vi "__createNewRoom.vi"(11 "room_name":string) -> (2 "new_room":T1, 3 "room_id":string)   [LabVIEW 2020, in "Room-API.lvclass"]
uses:
  Room-API.lvclass
  Single Room.ctl
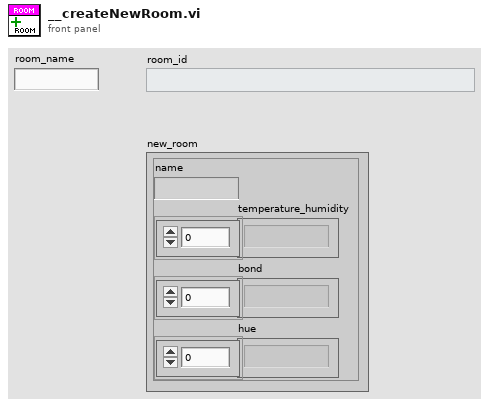
[diagram p1: front panel]
types:
  T1 = typedef "Room-API.lvclass/Single Room.ctl" = cluster{"name":string, "temperature_humidity":string[], "bond":string[], "hue":string[]}
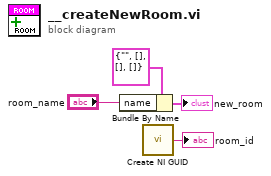
[diagram p0: block diagram]
diagram:
  n1 = Bundle By Name(cluster=T1 {"name"="", "temperature_humidity"=[], "bond"=[], "hue"=[]} ("singleRoom"), "name"="room_name") -> (→"new_room":T1)
  n2 = call <vilib>:"Create NI GUID.vi"() -> ("NI GUID"=→"room_id":string)
